vi "Write Direction.vi"(8 "error in (no error)":errorcluster, 10 "Direction":T1, 11 "Awesome! in":refnum<class "Awesome!.lvclass">) -> (0 "error out":errorcluster, 3 "Awesome! out":refnum<class "Awesome!.lvclass">)   [LabVIEW 2016, in "Awesome!.lvclass"]
uses:
  Awesome!.lvclass
  Type Defs/Direction Enum.ctl
  Awesome!.lvclass/Awesome!.ctl
  Type Defs/SB Type Defs.lvlib
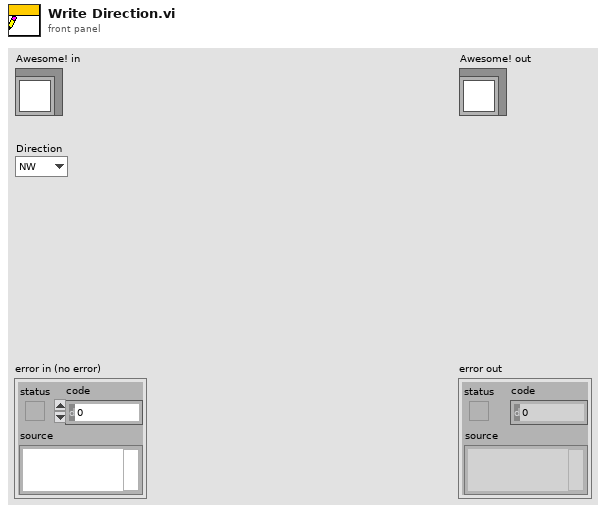
[diagram p1: front panel]
types:
  T1 = typedef "SB Type Defs.lvlib/Direction Enum.ctl" = enum16{"NW", "N", "NE", "E", "SE", "S", "SW", "W"}
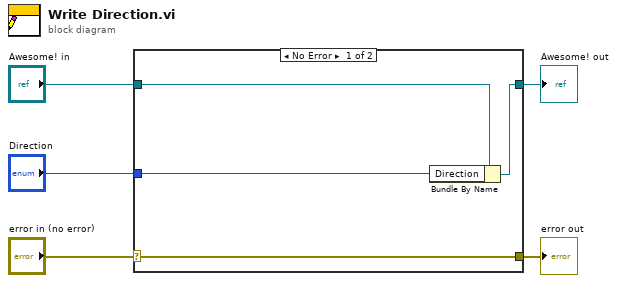
[diagram p0: block diagram]
diagram:
  n1 = case shown="No Error" "error in (no error)" {
    selector: "error in (no error)" -> [w9 w10]
    tunnel: [w9 w10] -> w4
    tunnel: [w7 w11] -> w2
    tunnel: "Awesome! in" -> [w8 w11]
    tunnel: "Direction" -> [w6 _]
    frame No Error {
      n2 = Bundle By Name(cluster=w8, "Direction"=w6) -> (w7:refnum<class "Awesome!.lvclass">)
    }
    frame Error {
    }
  }
  "error out" <- w4
  "Awesome! out" <- w2
